vi "Generate Scan Coordinates.vi"(7 "Scan Pattern":T1(ring), 10 "Y Axis":T2, 11 "X Axis":T2) -> (1 "Array":cluster{"X":dbl, "Y":dbl}[](array[cluster]), 2 "Y Scale":dbl[](array[numeric]), 3 "X Scale":dbl[](array[numeric]), 5 "# X tiles":i32)   [LabVIEW 2018]
uses:
  <vilib>/Analysis/1siggen.llb/Ramp Pattern by Samples.vi
  <vilib>/Analysis/NI_AALBase.lvlib
panel:
  out "XY Graph":cluster{"X":dbl, "Y":dbl}[](graph)
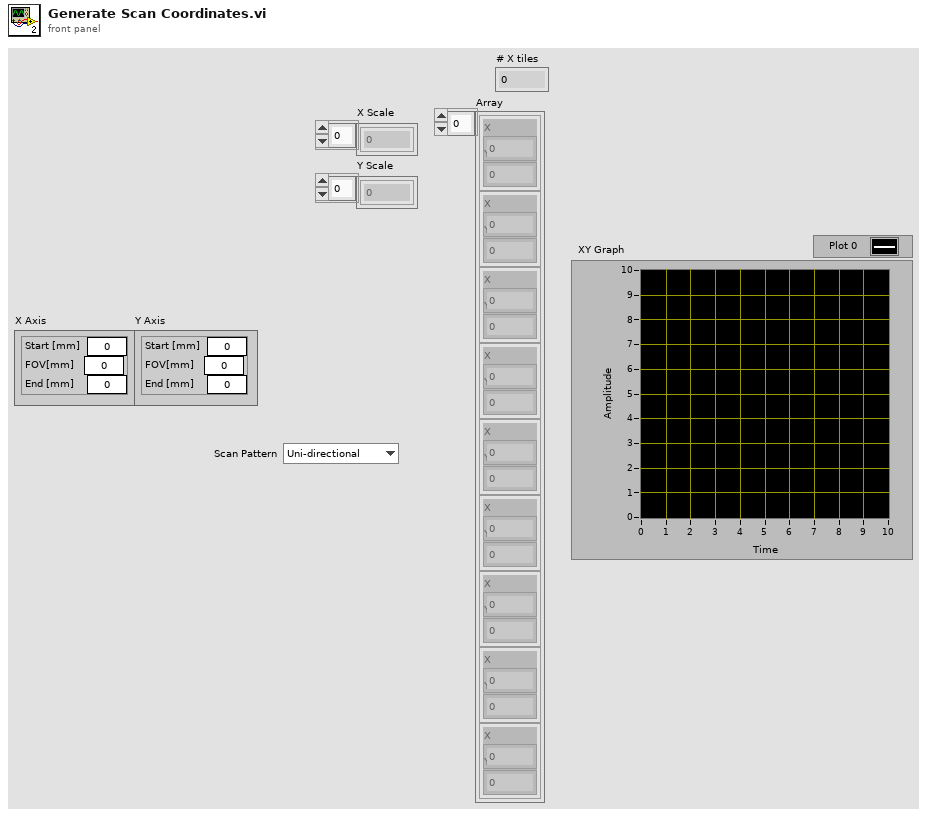
[diagram p1: front panel]
types:
  T1 = enum16{"Uni-directional", "Bi-Directional", "Spiral Out", "Spiral In"}
  T2 = cluster{"Start [mm]":dbl, "FOV[mm]":dbl, "End [mm]":dbl}
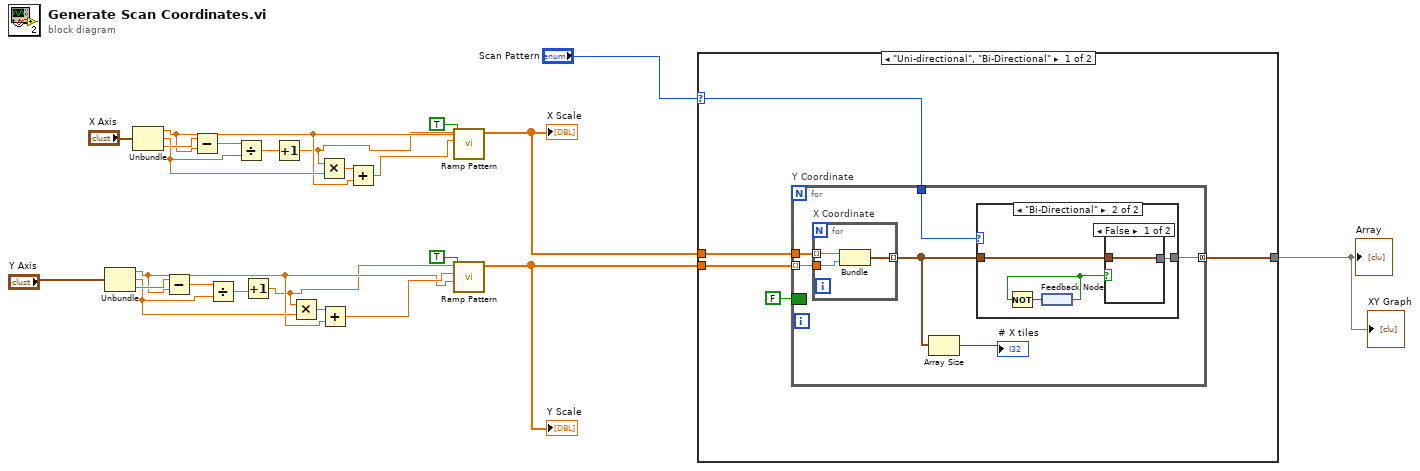
[diagram p0: block diagram]
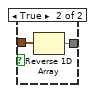
[diagram p3: hidden frame]
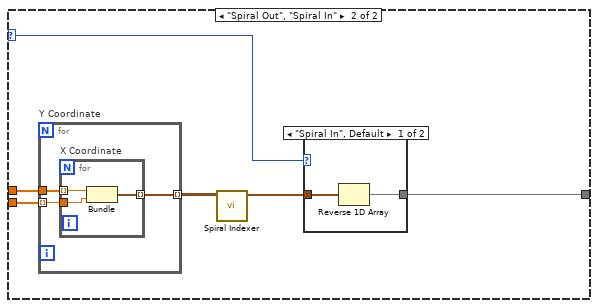
[diagram p4: hidden frame]
diagram:
  n1 = Unbundle("Y Axis") -> ("Start [mm]"=w7:dbl, "FOV[mm]"=w11:dbl, "End [mm]"=w13:dbl)
  n2 = Unbundle("X Axis") -> ("Start [mm]"=w15:dbl, "FOV[mm]"=w17:dbl, "End [mm]"=w19:dbl)
  n3 = Subtract(x=w13, y=w7) -> (x-y=w12:dbl)
  n4 = Subtract(x=w19, y=w15) -> (x-y=w18:dbl)
  n5 = Divide(x=w12, y=w11) -> (x/y=w2:dbl)
  n6 = Divide(x=w18, y=w17) -> (x/y=w6:dbl)
  n7 = Increment(x=w2) -> (x+1=w1:dbl)
  n8 = Increment(x=w6) -> (x+1=w5:dbl)
  n9 = Multiply(x=w1, y=w11) -> (x*y=w10:dbl)
  n10 = Multiply(x=w5, y=w17) -> (x*y=w16:dbl)
  n11 = Add(x=w10, y=w7) -> (x+y=w8:dbl)
  n12 = Add(x=w16, y=w15) -> (x+y=w14:dbl)
  n13 = call-poly <vilib>:"Ramp Pattern.vi"("exclude end?"=TRUE, "start"=w15, "end"=w14, "samples"=w5) -> ("Ramp Pattern"=w23:dbl[])  [unwired: 6 in, 1 out]
  "X Scale" <- w23
  n14 = call-poly <vilib>:"Ramp Pattern.vi"("exclude end?"=TRUE, "start"=w7, "end"=w8, "samples"=w1) -> ("Ramp Pattern"=w22:dbl[])  [unwired: 6 in, 1 out]
  "Y Scale" <- w22
  n15 = case shown="\"Uni-directional\", \"Bi-Directional\"" "Scan Pattern" {
    selector: "Scan Pattern" -> [w25 w49]
    tunnel: w23 -> [w29 w52]
    tunnel: w22 -> [w28 w51]
    tunnel: [w27 w48] -> w20
    frame "Uni-directional", "Bi-Directional" {
      n16 = for "Y Coordinate" {
        tunnel: w29 -> [w35]
        tunnel: w28 -> [w34] mode=indexing
        tunnel: [w32] -> w27 mode=concatenating
        tunnel: w25 -> [w33]
        border: FALSE -> [_]
        n17 = for "X Coordinate" {
          tunnel: w35 -> [w46] mode=indexing
          tunnel: w34 -> [w45]
          tunnel: [w44] -> w31 mode=indexing
          n18 = Bundle(w46, w45) -> (w44:cluster{dbl, dbl})  [unwired: 1 in]
        }
        n19 = Array Size(array=w31) -> (size(s)=→"# X tiles":i32)
        n20 = case shown="\"Bi-Directional\"" w33 {
          tunnel: w31 -> [w36 w38]
          tunnel: [w36 w39] -> w32
          frame "Uni-directional", Default {
          }
          frame "Bi-Directional" {
            n21 = feedback #1() -> (w37:bool)
            n22 = Not(x=w37) -> (.not. x?=w40:bool)
            n23 = feedback-in #1(w40) -> ()
            n24 = case shown="False" w37 {
              tunnel: [w41 w43] -> w39
              tunnel: w38 -> [w41 w42]
              frame False {
              }
              frame True {
                n25 = Reverse 1D Array(array=w42) -> (reversed array=w43:cluster{dbl, dbl}[])
              }
            }
          }
        }
      }
    }
    frame "Spiral Out", "Spiral In" {
      n26 = for "Y Coordinate" {
        tunnel: w52 -> [w58]
        tunnel: w51 -> [w57] mode=indexing
        tunnel: [w56] -> w50 mode=indexing
        n27 = for "X Coordinate" {
          tunnel: w58 -> [w61] mode=indexing
          tunnel: w57 -> [w60]
          tunnel: [w59] -> w56 mode=indexing
          n28 = Bundle(w61, w60) -> (w59:cluster{dbl, dbl})  [unwired: 1 in]
        }
      }
      n29 = call "Spiral Indexer.vi"("Array 2"=w50) -> ("Array"=w47:cluster{dbl, dbl}[])  [unwired: 10 in]
      n30 = case shown="\"Spiral In\", Default" w49 {
        tunnel: [w53 w55] -> w48
        tunnel: w47 -> [w54 w55]
        frame "Spiral In", Default {
          n31 = Reverse 1D Array(array=w54) -> (reversed array=w53:cluster{dbl, dbl}[])
        }
        frame "Spiral Out" {
        }
      }
    }
  }
  "Array" <- w20
  "XY Graph" <- w20
